vi "rapid_make_traces.vi"(9 "Time":dbl[](array[numeric]), 10 "Channel B":dbl[][](array[numeric]), 11 "Channel A":dbl[][](array[numeric])) -> (2 "Channel B Out":dbl[][][](array[numeric]), 3 "Channel A Out":dbl[][][](array[numeric]))   [LabVIEW 2016]
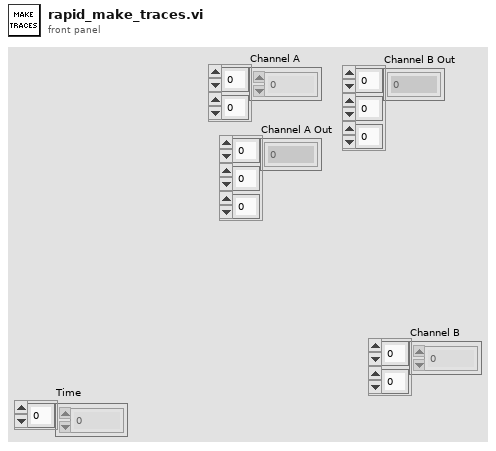
[diagram p1: front panel]
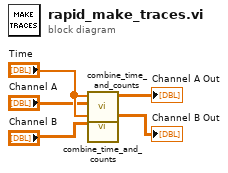
[diagram p0: block diagram]
diagram:
  n1 = call "combine_time_and_counts.vi"("Voltage In"="Channel A", "Time"="Time") -> ("Traces Out"=→"Channel A Out":dbl[][][])  [unwired: 9 in]
  n2 = call "combine_time_and_counts.vi"("Voltage In"="Channel B", "Time"="Time") -> ("Traces Out"=→"Channel B Out":dbl[][][])  [unwired: 9 in]
